vi "DSP Enqueue.vi"(8 "error in (no error)":errorcluster, 11 "Sample Buffer":u8[](array[numeric])) -> (0 "error out":errorcluster)   [LabVIEW 2016]
uses:
  <vilib>/rvi/interface/nirviMethod/nirviMethod.xnode
  FPGA Control/FPGA Global Variables.vi
  <vilib>/FPGAPlugInAG/Dynamic/niLvFpga_WriteFifo_Dynamic.vi
  <vilib>/rvi/errors/niLvFpgaMergeErrorWithErrorCode.vi
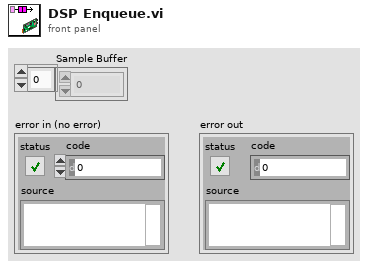
[diagram p1: front panel]
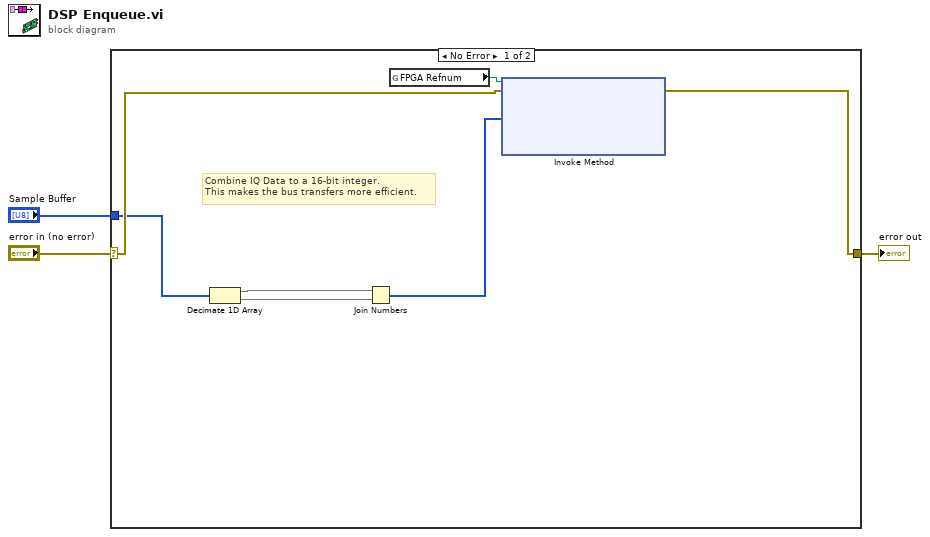
[diagram p0: block diagram]
diagram:
  n1 = case shown="No Error" "error in (no error)" {
    selector: "error in (no error)" -> [w7 w11]
    tunnel: "Sample Buffer" -> [w6 _]
    tunnel: [w5 w11] -> w3
    frame No Error {
      # "Combine IQ Data to a 16-bit integer.\nThis makes the bus transfers more efficient."
      n2 = Decimate 1D Array(w6) -> (w9:u8[], w10:u8[])
      n3 = Join Numbers(hi=w9, lo=w10) -> ((hi.lo)=w4:u16[])
      n4 = global read "FPGA Global Variables.vi" "FPGA Refnum"() -> (w8:refnum<k20>)
      n5 = xnode "Invoke Method"("FPGA VI Reference In"=w8, "error in"=w7, "Data"=w4) -> ("error out"=w5:errorcluster)  [unwired: 1 in, 2 out]
    }
    frame Error {
    }
  }
  "error out" <- w3
